vi "OpenCOM.vi"(0 "VISA resource name":refnum<visa-resource-name>, 1 "baud rate (9600)":u32=9600, 2 "data bits":u16=8 min=5 max=8 step=1, 3 "parity":u16(ring) items=["None", "Odd", "Even", "Mark", "Space"], 4 "stop bits":u16(ring)=10 items=["1.0"=10, "1.5"=15, "2.0"=20], 5 "flow control":u16(ring) items=["None"=0, "XON/XOFF"=1, "RTS/CTS"=2, "DTR/DSR"=4], 6 "termination char\n(0xA = '\\n' = LF)":u8=10 format="%.0x", 7 "timeout(ms) solitamente 50ms":u32=10000, 13 "End Write termination character?":bool=TRUE, 17 "End read on termination character?":bool=TRUE) -> (20 "VISA resource name out":refnum<visa-resource-name>, 27 "error out":errorcluster)   [LabVIEW 2019]
uses:
  <vilib>/Instr/_visa.llb/VISA Configure Serial Port (Instr).vi
panel:
  in  "error out 2":errorcluster
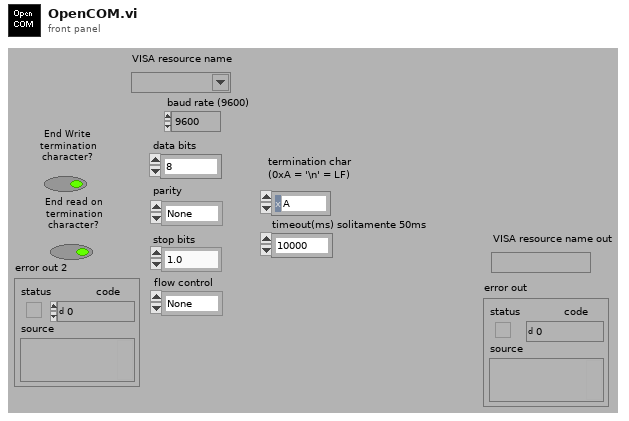
[diagram p1: front panel]
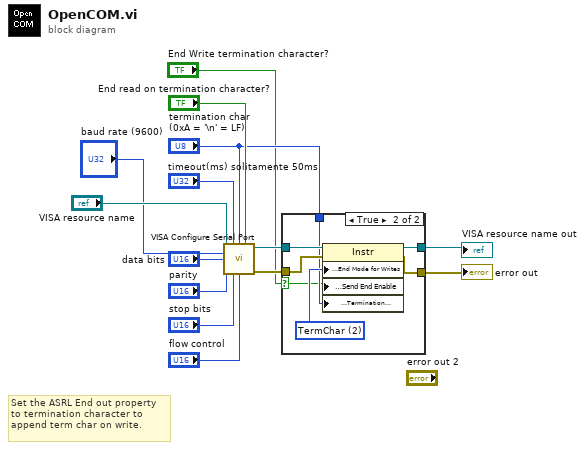
[diagram p0: block diagram]
diagram:
  # "Set the ASRL End out property\nto termination character to\nappend term char on write."
  n1 = call-poly "VISA Configure Serial Port"("VISA resource name"="VISA resource name", "timeout (10sec)"="timeout(ms) solitamente 50ms", "termination char\n(0xA = '\\n' = LF)"="termination char\n(0xA = '\\n' = LF)", "Enable Termination\nChar (T)"="End read on termination character?", "baud rate (9600)"="baud rate (9600)", "data bits (8)"="data bits", "parity (0:none)"="parity", "stop bits (10: 1 bit)"="stop bits", "flow control (0:none)"="flow control") -> ("VISA resource name out"=w6:refnum<visa-resource-name>, "error out"=w7:errorcluster)  [unwired: 1 in, 4 out]
  n2 = case shown="True" "End Write termination character?" {
    selector: "End Write termination character?" -> [_ w18]
    tunnel: w6 -> [w15 w23]
    tunnel: w7 -> [w16 w22]
    tunnel: [w15 w21] -> w3
    tunnel: [w16 w17] -> w4
    tunnel: "termination char\n(0xA = '\\n' = LF)" -> [_ w19]
    frame False {
    }
    frame True {
      w20 = u16 2 items=["None", "LastBit", "TermChar", "Break"] ("Serial Settings:Serial End Mode for Writes")
      n3 = property class="Instr"(reference=w23, error in=w22, "Serial Settings:End Mode for Writes"=w20, "Message Based Settings:Send End Enable"=w18, "Message Based Settings:Termination Character"=w19) -> (reference out=w21:refnum<visa-resource-name>, error out=w17:errorcluster)
    }
  }
  "error out" <- w4
  "VISA resource name out" <- w3
